vi "database platform path.vi"(11 "database":string="database1") -> (3 "Path out":string)   [LabVIEW 2016]
uses:
  Access/Access Lib.lvlib
  SQLite/SQLite Lib.lvlib
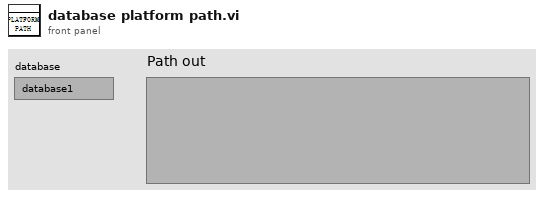
[diagram p1: front panel]
types:
  T1 = typedef "数据库类型.ctl" = enum16{"Access", "SQLite"}
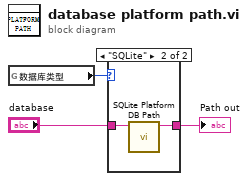
[diagram p0: block diagram]
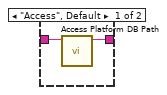
[diagram p2: hidden frame]
diagram:
  n1 = global read "外部调用接口全局变量.vi" "数据库类型"() -> (w1:T1)
  n2 = case shown="\"SQLite\"" w1 {
    tunnel: [w5 w7] -> w2
    tunnel: "database" -> [w4 w6]
    frame "Access", Default {
      n3 = call "Access Platform DB Path.vi"("名称或相对路径"=w4) -> ("Path out"=w5:string)  [unwired: 9 in, 1 out]
    }
    frame "SQLite" {
      n4 = call "SQLite Platform DB Path.vi"("名称或相对路径"=w6) -> ("Path out"=w7:string)  [unwired: 10 in]
    }
  }
  "Path out" <- w2
